vi "Unsafely Disintegrate.vi"(11 "Bricks in":T1(array[cluster])) -> (3 "Total Disintegrated":u64)   [LabVIEW 2023, in "d22.lvlib"]
uses:
  d22.lvlib
  f063d734-7f55-4156-8ebd-3168d71ec41a.vi
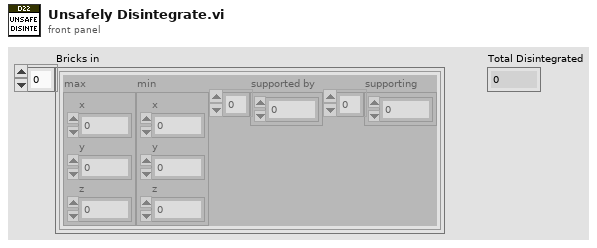
[diagram p1: front panel]
types:
  T1 = cluster{"max":cluster{"x":i32, "y":i32, "z":i32}, "min":cluster{"x":i32, "y":i32, "z":i32}, "supported by":i32[], "supporting":i32[]}[]
  T2 = cluster{"max":cluster{"x":i32, "y":i32, "z":i32}, "min":cluster{"x":i32, "y":i32, "z":i32}, "supported by":i32[], "supporting":i32[]}
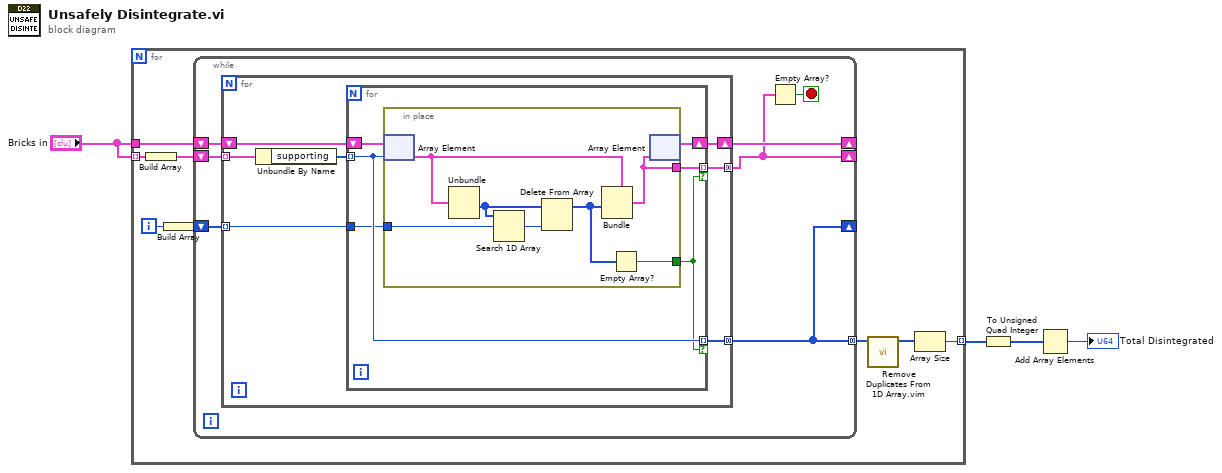
[diagram p0: block diagram]
diagram:
  n1 = for {
    tunnel: "Bricks in" -> [w8] mode=indexing
    tunnel: "Bricks in" -> [w9]
    tunnel: [w10] -> w4 mode=indexing
    i -> [w6]
    n2 = Build Array(w8) -> (w7:T1)
    n3 = Build Array(w6) -> (w5:i32[])
    n4 = while {
      shift-right: [w15] -> _
      shift-left: w7 -> [w19]
      tunnel: [w14] -> w12 mode=concatenating
      shift-right: [w16] -> _
      shift-left: w9 -> [w18]
      shift-right: [w14] -> _
      shift-left: w5 -> [w13]
      stop <- w17 stop-if-true
      n5 = for {
        tunnel: w19 -> [w26] mode=indexing
        tunnel: [w22] -> w14 mode=concatenating
        shift-right: [w23] -> w16
        shift-left: w18 -> [w25]
        tunnel: [w21] -> w15 mode=concatenating
        tunnel: w13 -> [w20] mode=indexing
        n6 = Unbundle By Name(w26) -> ("supporting"=w24:i32[])
        n7 = for {
          tunnel: w24 -> [w30] mode=indexing
          shift-right: [w31] -> w23
          shift-left: w25 -> [w32]
          tunnel: [w30] -> w22 mode=indexing if=w28
          tunnel: [w29] -> w21 mode=indexing if=w28
          tunnel: w20 -> [w27]
          n8 = in-place {
            in-place-border: [w35] -> w28
            in-place-border: [w34] -> w29
            in-place-border: w27 -> [w33]
            n9 = in-place-array #1(w32, w30) -> (w39:T2)
            n10 = Unbundle(w39) -> ("supported by"=w37:i32[])  [unwired: 3 out]
            n11 = Search 1D Array(1D array=w37, element=w33) -> (index of element=w38:i32)  [unwired: 1 in]
            n12 = Delete From Array(array=w37, index=w38) -> (array with subset deleted=w36:i32[])  [unwired: 1 in, 1 out]
            n13 = Bundle(cluster=w39, "supported by"=w36) -> (w34:T2)  [unwired: 3 in]
            n14 = Empty Array?(array=w36) -> (empty?=w35:bool)
            n15 = in-place-array #1(w34) -> (w31:T1)  [unwired: 1 out]
          }
        }
      }
      n16 = Empty Array?(array=w15) -> (empty?=w17:bool)
    }
    n17 = call "Remove Duplicates From 1D Array.vim"("array"=w12) -> ("array with duplicates removed"=w11:i32[])  [unwired: 10 in]
    n18 = Array Size(array=w11) -> (size(s)=w10:i32)
  }
  n19 = To Unsigned Quad Integer(1:w4) -> (0:w2:u64[])
  n20 = Add Array Elements(numeric array=w2) -> (sum=→"Total Disintegrated":u64)
